vi "Close section.vi"(8 "error in (no error)":errorcluster, 11 "Plain Text Report In":refnum<class "Plain Text Report.lvclass">) -> (0 "error out":errorcluster, 3 "Plain Text Report Out":refnum<class "Plain Text Report.lvclass">)   [LabVIEW 2020, in "Plain Text Report.lvclass"]
uses:
  Plain Text Report.lvclass
  Plain Text Report.lvclass/Plain Text Report.ctl
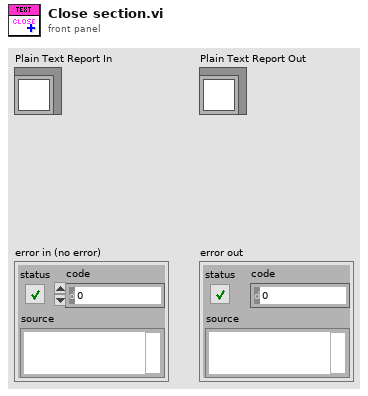
[diagram p1: front panel]
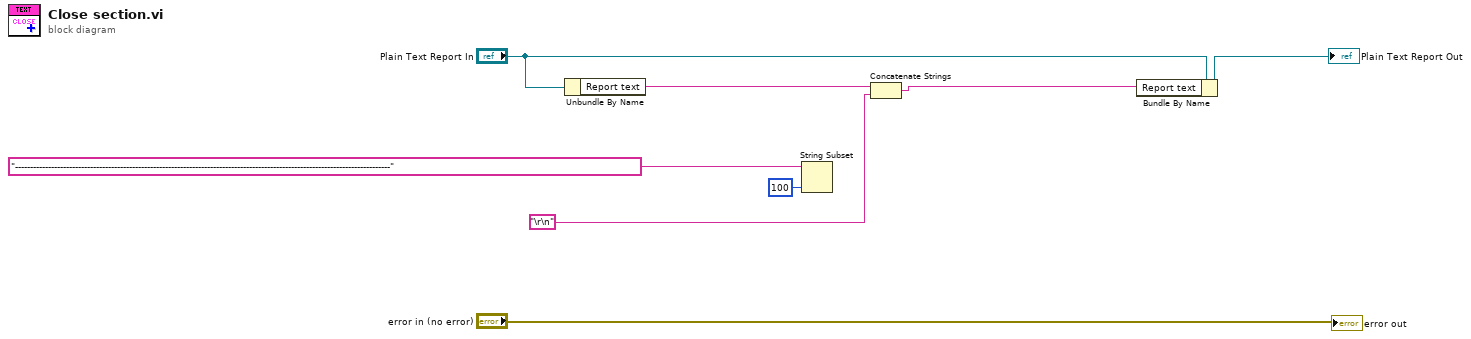
[diagram p0: block diagram]
diagram:
  n1 = Unbundle By Name("Plain Text Report In") -> ("Report text"=w2:string)
  n2 = String Subset(string="-----------------------------------------------------------------------------------------------------------------------------" ("format string"), length (rest)=100 ("length (rest)")) -> ()  [unwired: 1 in, 1 out]
  n3 = Concatenate Strings(w2, "\r\n") -> (w3:string)
  n4 = Bundle By Name(cluster="Plain Text Report In", "Report text"=w3) -> (→"Plain Text Report Out":refnum<class "Plain Text Report.lvclass">)
  "error out" <- "error in (no error)"
